vi "testFgenBasic.vi"() -> ()   [LabVIEW 2023]
doc: "<b>Author:</b> Wolfgang\n<b>Description:</b> Basic Arb/Fgen abstraction test"
uses:
  Data/arbType.ctl
  Data/arbWaveformType.ctl
  Arb.lvclass
  sweArb.lvlib
panel:
  out "error out":errorcluster
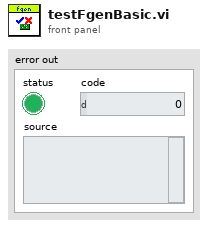
[diagram p1: front panel]
types:
  T1 = typedef "sweArb.lvlib/arbWaveformType.ctl" = enum16{"Sine", "Square", "Triangle", "DC", "Noise", "Arb"}
  T2 = typedef "sweArb.lvlib/arbType.ctl" = enum16{"Simulated", "FGEN_NI", "FGEN_Keysight"}
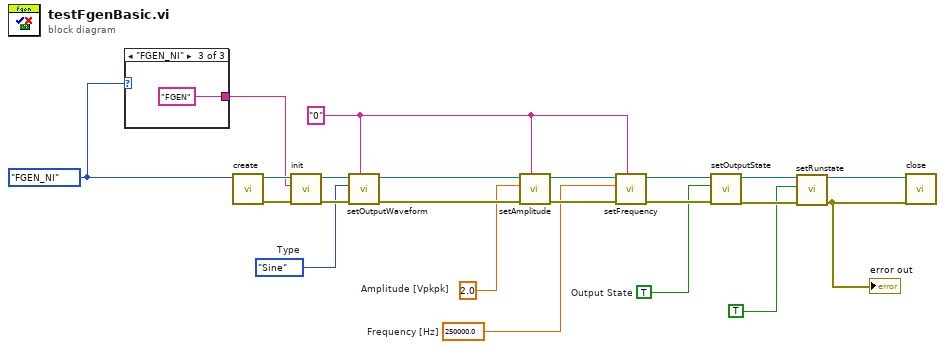
[diagram p0: block diagram]
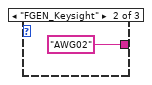
[diagram p3: hidden frame]
diagram:
  w7 = 250000.0  # Frequency [Hz]
  w8 = TRUE  # Output State
  w10 = 2.0  # Amplitude [Vpkpk]
  w11 = arbWaveformType."Sine"  # Type
  w9 = "0" ("Channel")
  w6 = arbType."FGEN_NI" ("Type")
  n1 = case shown="\"FGEN_NI\"" w6 {
    tunnel: [_ "AWG02" ("Resource") "FGEN" ("Resource")] -> w21
    frame "Simulated", Default {
    }
    frame "FGEN_Keysight" {
    }
    frame "FGEN_NI" {
    }
  }
  n2 = call "create.vi"("Type"=w6) -> ("error out"=w20:errorcluster, "Fgen.lvclass"=w22:refnum<class "Arb.lvclass">)  [unwired: 9 in]
  n3 = call-dynamic "init.vi"("error in (no error)"=w20, "Resource"=w21, "Instrument in"=w22) -> ("error out"=w18:errorcluster, "Instrument out"=w19:refnum<class "Arb.lvclass">)  [unwired: 7 in]
  n4 = call-dynamic "setOutputWaveform.vi"("Channel"=w9, "error in (no error)"=w18, "Type"=w11, "Fgen in"=w19) -> ("error out"=w16:errorcluster, "Fgen out"=w17:refnum<class "Arb.lvclass">)  [unwired: 6 in]
  n5 = call-dynamic "setAmplitude.vi"("Channel"=w9, "error in (no error)"=w16, "Amplitude [Vpkpk]"=w10, "Fgen in"=w17) -> ("error out"=w14:errorcluster, "Fgen out"=w15:refnum<class "Arb.lvclass">)  [unwired: 6 in]
  n6 = call-dynamic "setFrequency.vi"("Channel"=w9, "error in (no error)"=w14, "Frequency [Hz]"=w7, "Fgen in"=w15) -> ("error out"=w12:errorcluster, "Fgen out"=w13:refnum<class "Arb.lvclass">)  [unwired: 6 in]
  n7 = call-dynamic "setOutputState.vi"("error in (no error)"=w12, "Output State"=w8, "Fgen in"=w13) -> ("error out"=w4:errorcluster, "Fgen out"=w5:refnum<class "Arb.lvclass">)  [unwired: 7 in]
  n8 = call-dynamic "setRunstate.vi"("error in (no error)"=w4, "Runstate"=TRUE, "Fgen in"=w5) -> ("error out"=w1:errorcluster, "Fgen out"=w3:refnum<class "Arb.lvclass">)  [unwired: 7 in]
  "error out" <- w1
  n9 = call-dynamic "close.vi"("error in (no error)"=w1, "Instrument in"=w3) -> ()  [unwired: 9 in, 1 out]
